vi "Teleop.vi"(10 "Match Info":T7={"Autonomous Elapsed Seconds"=0.0, "TeleOp Elapsed Seconds"=0.0, "Disabled Elapsed Seconds"=0.0, "Visited Autonomous"=FALSE, "Visited TeleOp"=FALSE, "Visited Disabled"=FALSE, "Autonomous Settings"={"Autonomous Style"=enum."Independent", "VI Refnum"=refnum}}, 11 "Call Context":T8) -> ()   [LabVIEW 2018]
doc: "This VI is called for each TeleOp packet received from the DS where the robot is not disabled. It is often used to read from the joysticks and update I/O or to update setpoints for timed control loops. It should complete and return within 20 milliseconds or it may miss DS packets."
uses:
  <vilib>/Rock Robotics/WPI/DriverStation/WPI_DriverStationDerivedRobotMode.ctl
  <vilib>/Rock Robotics/WPI/DriverStation/WPI_DriverStationMatch Info.ctl
  <vilib>/Rock Robotics/WPI/ThirdParty/Phoenix-LabVIEW/Motor Controller/Controls/CTRE_Phoenix_MotorControl_ControlMode.ctl
  <vilib>/Rock Robotics/WPI/Solenoid/WPI_SolenoidValue.ctl
  <vilib>/Rock Robotics/WPI/Utilities/WPI_GetSetVariantRefNum.vi
  <vilib>/Rock Robotics/Network Tables/NT Write Boolean Array.vi
  <vilib>/Rock Robotics/Network Tables/NT Write Numeric Array.vi
  <vilib>/Rock Robotics/Network Tables/NT Read Boolean.vi
  <vilib>/Rock Robotics/Network Tables/NT Read Number.vi
  <vilib>/Rock Robotics/WPI/Solenoid/WPI_SolenoidSetEnum.vi
  <vilib>/Rock Robotics/WPI/ThirdParty/Phoenix-LabVIEW/Motor Controller/Get/CTRE_Phoenix_MotorController_GetSelectedSensorData.vi
  <vilib>/Utility/inputDevices.llb/joystickAcquire.vi
panel:
  in  "Cluster":T1={"Elevator Setpoints"=[0.0, 100000.0, 250000.0, 250000.0, 270000.0, 475000.0, 50000.0], "Wrist Setpoints"=[180000.0, 7600.0, 82000.0, 100000.0, 4000.0, 69000.0, 100000.0, 110000.0, 205000.0], "Horse Drive Setpoints"=[90000.0, 90000.0, 90000.0, 180000.0], "Wrist Gains"={"proportional gain (Kc)"=-1e-05, "integral time (Ti, min)"=0.01, "derivative time (Td, min)"=0.0}, "Wrist Power Limits"={"output high"=0.75, "output low"=-0.75}, "Horse Gains"={"proportional gain (Kc)"=1e-05, "integral time (Ti, min)"=0.02, "derivative time (Td, min)"=0.0}, "Horse Power Limits"={"output high"=0.25, "output low"=-0.25}, "Elevator Gains"={"proportional gain (Kc)"=1e-05, "integral time (Ti, min)"=0.01, "derivative time (Td, min)"=0.0}, "Elevator Power Limits"={"output high"=0.25, "output low"=-0.25}}
  in  "Wrist Manual Power":dbl step=0.05 format="%#_13g"
  in  "Elevator Manual Power":dbl step=0.05 format="%#_13g"
  in  "Elevator Level Select":T2(ring)
  in  "Horse Drive":T3(ring)
  in  "Wrist":T4(ring)
  in  "Climb Mode":bool
  in  "Elevator Switch":bool=TRUE
  in  "Enable Auto":bool=TRUE
  out "Intake Wrist Encoder":i32
  in  "Reset Intake Wrist":bool
  out "Horse Encoder":i32
  in  "Reset Horse Encoder":bool
  in  "Reset Elevator Encoder":bool
  out "Elevator Encoder":i32
  in  "ScoreMode 2":T5(ring)
  in  "Override Vision":bool
  out "element 2":T6
  in  "Butterfly Status":bool
  in  "ScoreMode":T5(ring)
  out "Sample Slider 0":dbl(slide) scale=0.0..5.0
  out "Sample Boolean 1":bool
  out "Sample Boolean 0":bool
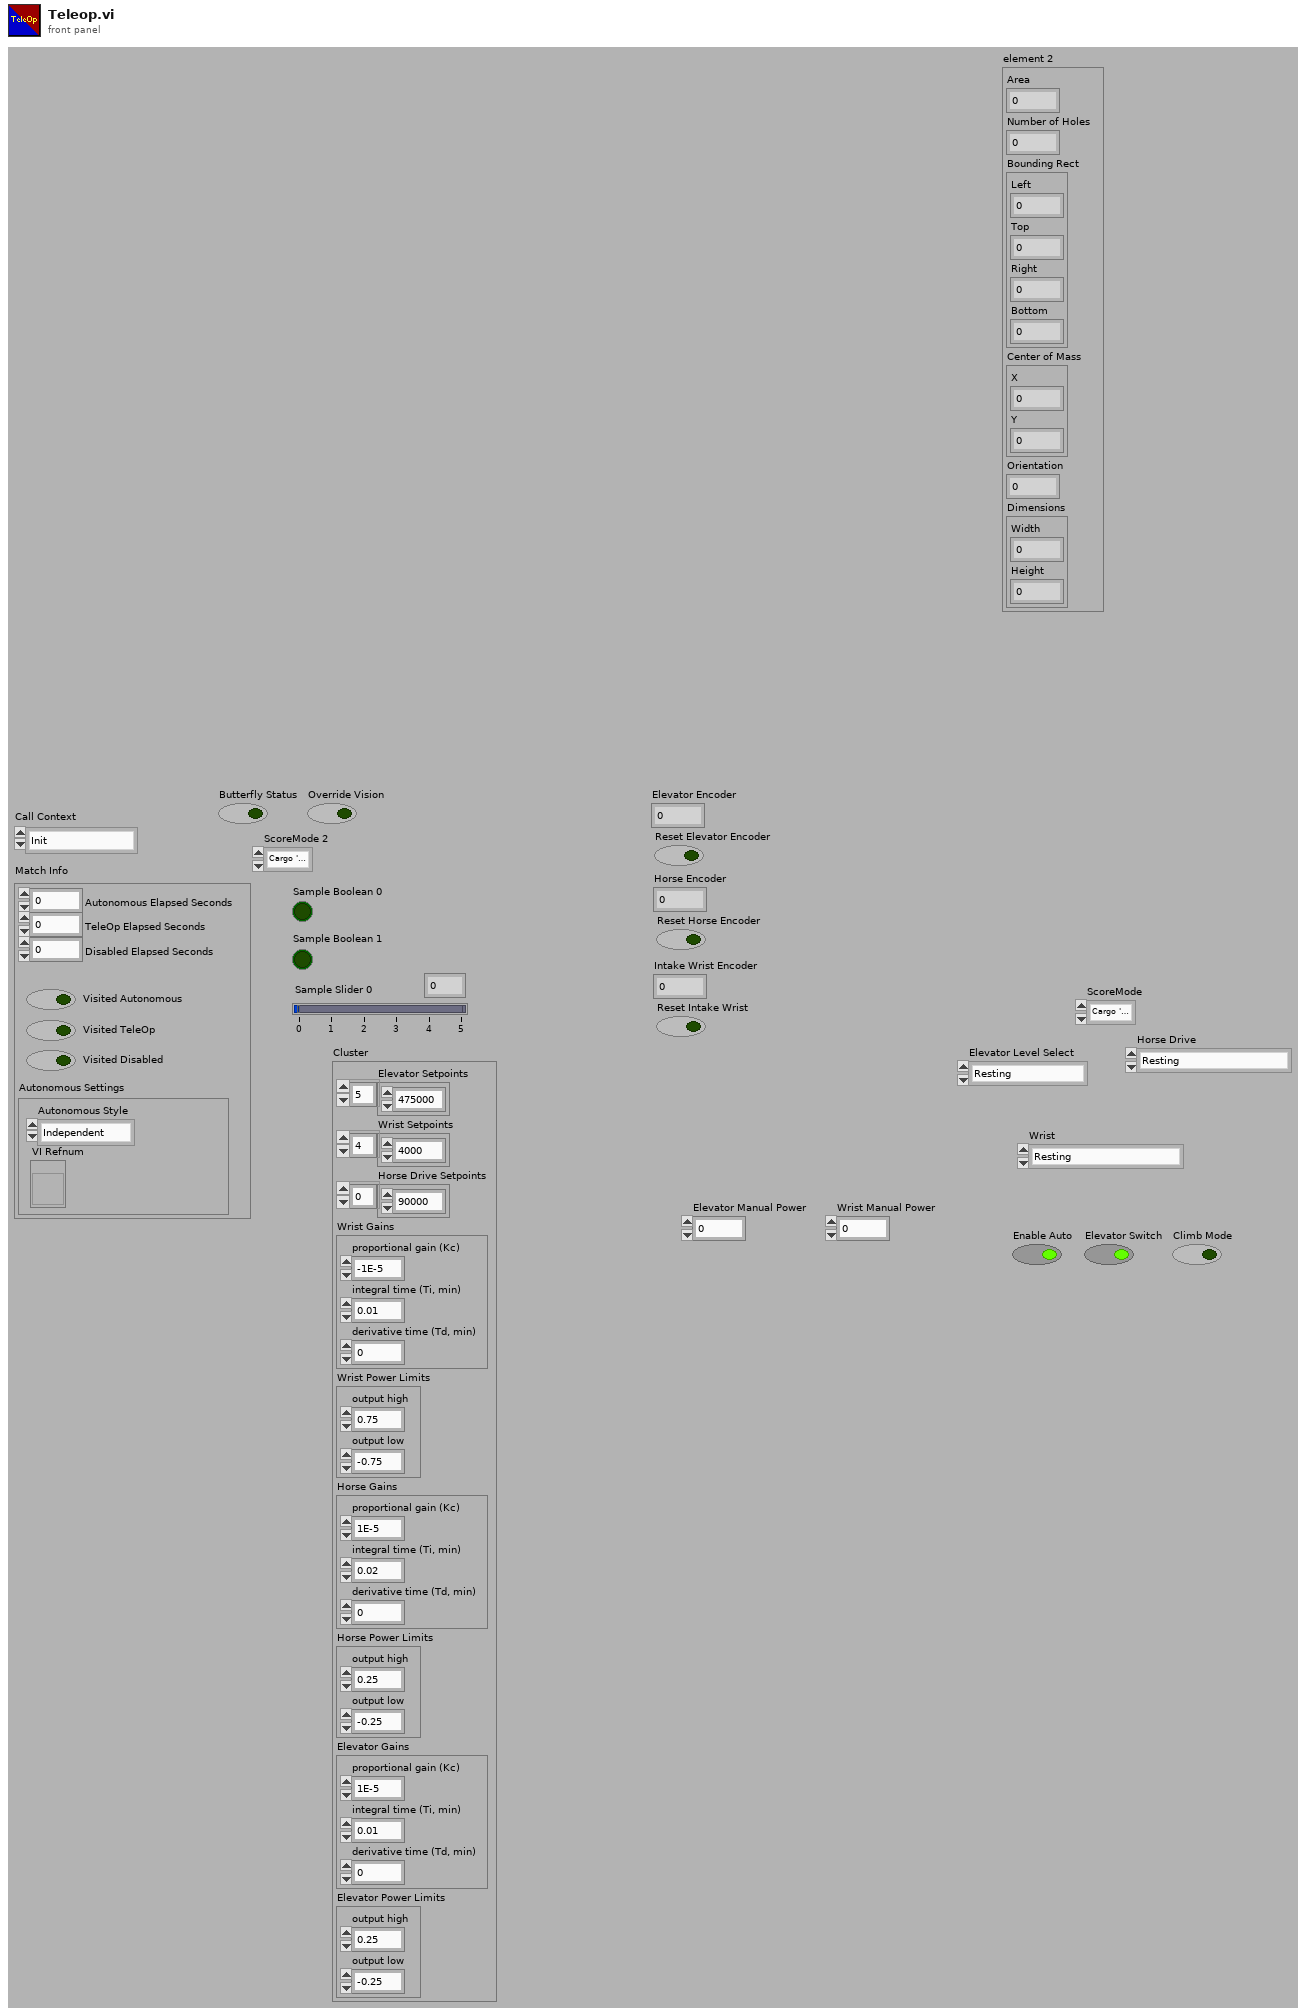
[diagram p1: front panel]
types:
  T1 = cluster{"Elevator Setpoints":dbl[], "Wrist Setpoints":dbl[], "Horse Drive Setpoints":dbl[], "Wrist Gains":cluster{"proportional gain (Kc)":dbl, "integral time (Ti, min)":dbl, "derivative time (Td, min)":dbl}, "Wrist Power Limits":cluster{"output high":dbl, "output low":dbl}, "Horse Gains":cluster{"proportional gain (Kc)":dbl, "integral time (Ti, min)":dbl, "derivative time (Td, min)":dbl}, "Horse Power Limits":cluster{"output high":dbl, "output low":dbl}, "Elevator Gains":cluster{"proportional gain (Kc)":dbl, "integral time (Ti, min)":dbl, "derivative time (Td, min)":dbl}, "Elevator Power Limits":cluster{"output high":dbl, "output low":dbl}}
  T2 = enum16{"Resting", "CargoShip Front", "CargoShip Back", "Cargo Mid", "Hatch Mid", "All High", "Cargo Intake"}
  T3 = enum16{"Resting", "PLACEHOLDER", "Hatch Intake", "Lift"}
  T4 = enum16{"Resting", "Hatch Ground Intake", "Hatch Place Low/Mid/CargoShip", "Hatch Place High", "Cargo Ground Intake", "Cargo Place Low/Mid", "Cargo Place High", "CargoShip Place Front", "CargoShip Place Back"}
  T5 = enum16{"Cargo 'default'", "Hatch", "HorseDriveHatch"}
  T6 = cluster{"Area":dbl, "Number of Holes":dbl, "Bounding Rect":cluster{"Left":dbl, "Top":dbl, "Right":dbl, "Bottom":dbl}, "Center of Mass":cluster{"X":dbl, "Y":dbl}, "Orientation":dbl, "Dimensions":cluster{"Width":dbl, "Height":dbl}}
  T7 = typedef "WPI_DriverStationMatch Info.ctl" = cluster{"Autonomous Elapsed Seconds":dbl, "TeleOp Elapsed Seconds":dbl, "Disabled Elapsed Seconds":dbl, "Visited Autonomous":bool, "Visited TeleOp":bool, "Visited Disabled":bool, "Autonomous Settings":cluster{"Autonomous Style":enum16{"Iterative", "Independent"}, "VI Refnum":refnum<vi>}}
  T8 = typedef "WPI_DriverStationDerivedRobotMode.ctl" = enum16{"Init", "Execute", "Stop"}
  T9 = typedef "WPI_SolenoidValue.ctl" = enum16{"Off", "On", "Forward", "Reverse"}
  T10 = typedef "CTRE_Phoenix_MotorControl_ControlMode.ctl" = u16
  T11 = typedef "WPI_SolenoidDevRef.ctl" = cluster{"DevStatus":errorcluster, "Pneumatics Control Module":u8, "Forward Solenoid Channel":T12, "Reverse Solenoid Channel":T12}
  T12 = typedef "WPI_SolenoidChannel.ctl" = enum8{"Solenoid 0", "Solenoid 1", "Solenoid 2", "Solenoid 3", "Solenoid 4", "Solenoid 5", "Solenoid 6", "Solenoid 7", "Invalid"}
  T13 = typedef "WPI_JoystickDevRef.ctl" = cluster{"Device":T14}
  T14 = typedef "WPI_JoystickDeviceEnum.ctl" = enum16{"USB 0", "USB 1", "USB 2", "USB 3", "USB 4", "USB 5"}
  T15 = typedef "WPI_MotorControlDeviceRef.ctl" = cluster{"DeviceStatus":errorcluster, "Type":T16, "PWM":cluster{"PWM Channel":T17, "DeadBand":T18}, "CAN":cluster{"Device Number":u8, "SetOutput VI Ref":variant, "GetOutput VI Ref":variant, "Enable VI Ref":variant, "Disable VI Ref":variant, "Data":variant}, "Invert":bool, "DIO PWM":cluster{"PWM \"Enable\" Channel":T17, "DIOChannel":T19, "PWM Rate":dbl}}
  T16 = typedef "WPI_MotorControlType.ctl" = enum16{"PWM", "CAN", "DIO PWM"}
  T17 = typedef "FPGA_DIOPWMChannel.ctl" = enum8{"PWM 0", "PWM 1", "PWM 2", "PWM 3", "PWM 4", "PWM 5", "PWM 6", "PWM 7", "PWM 8", "PWM 9", "PWM MXP 0", "PWM MXP 1", "PWM MXP 2", "PWM MXP 3", "PWM MXP 4", "PWM MXP 5", "PWM MXP 6", "PWM MXP 7", "PWM MXP 8", "PWM MXP 9", "Invalid"}
  T18 = typedef "WPI_PWMDeadband.ctl" = cluster{"Name":string, "maxPositivePwm":i32, "minPositivePwm":i32, "centerPwm":i32, "maxNegativePwm":i32, "minNegativePwm":i32, "angularRange":u16}
  T19 = typedef "FPGA_DIOChannel.ctl" = enum8{"DIO 0", "DIO 1", "DIO 2", "DIO 3", "DIO 4", "DIO 5", "DIO 6", "DIO 7", "DIO 8", "DIO 9", "DIO MXP 0", "DIO MXP 1", "DIO MXP 2", "DIO MXP 3", "DIO MXP 4", "DIO MXP 5", "DIO MXP 6", "DIO MXP 7", "DIO MXP 8", "DIO MXP 9", "DIO MXP 10", "DIO MXP 11", "DIO MXP 12", "DIO MXP 13", "DIO MXP 14", "DIO MXP 15", "SPI Port CS1", "SPI Port CS2", "SPI Port CS3", "SPI Port MISO", "SPI Port MOSI", "Invalid"}
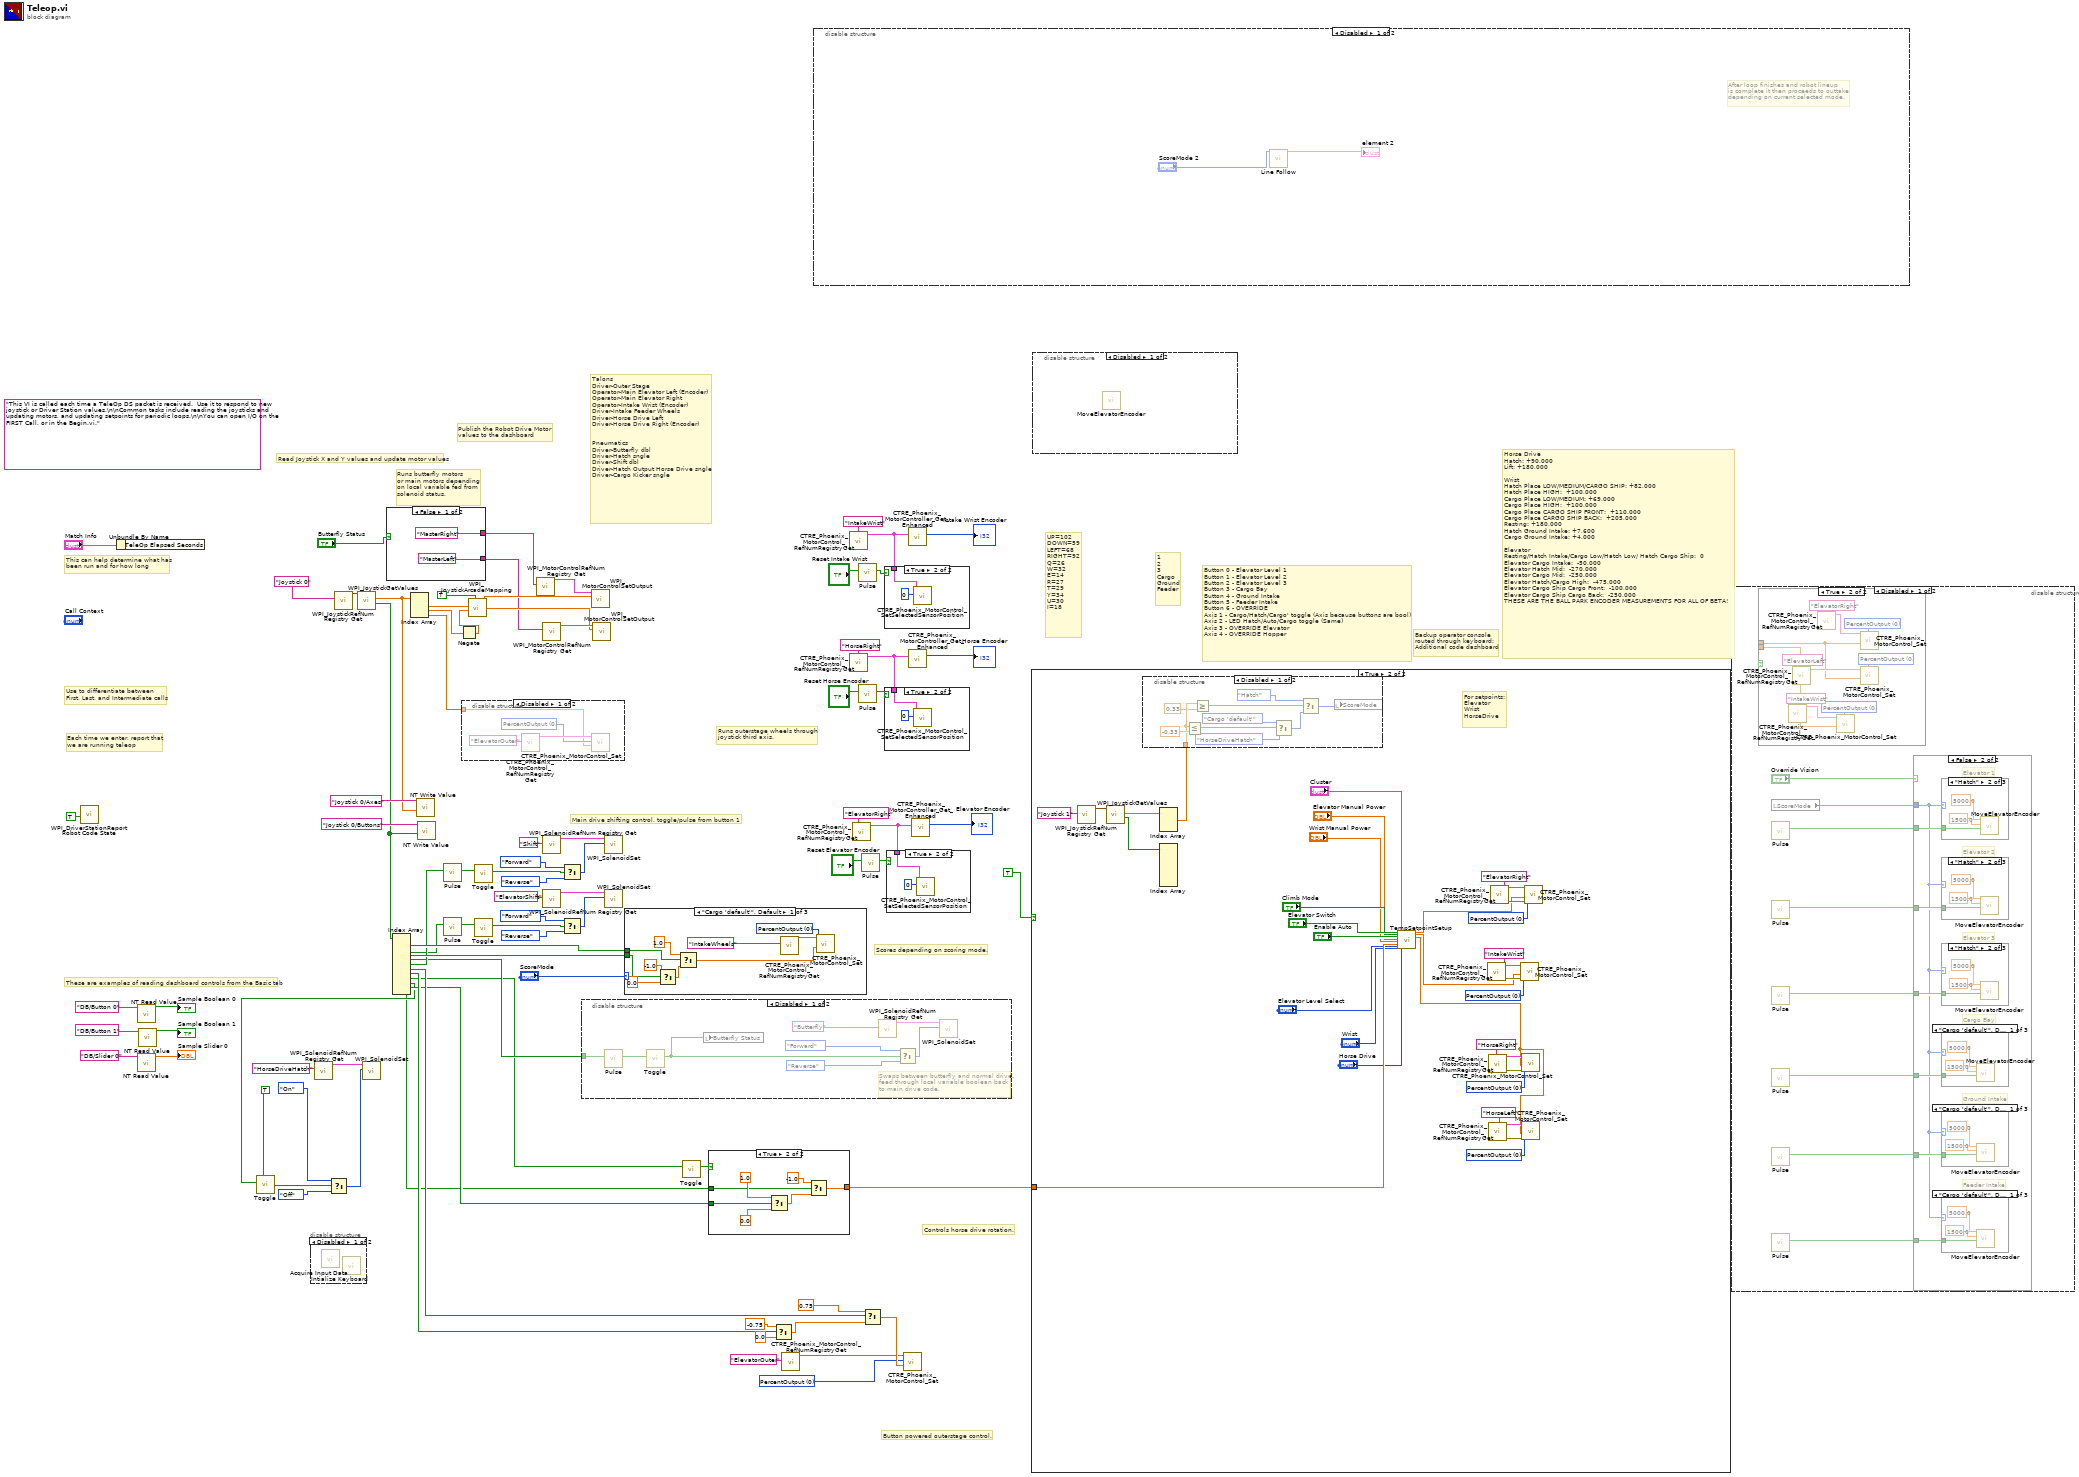
[diagram p0: block diagram]
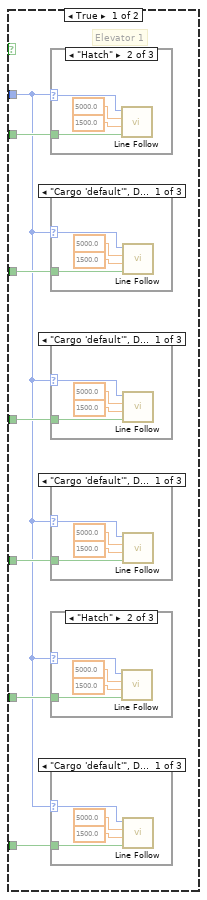
[diagram p3: hidden frame]
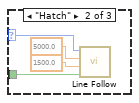
[diagram p4: hidden frame]
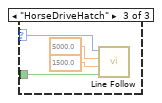
[diagram p5: hidden frame]
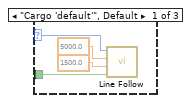
[diagram p6: hidden frame]
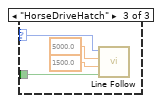
[diagram p7: hidden frame]
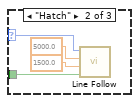
[diagram p8: hidden frame]
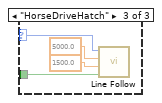
[diagram p9: hidden frame]
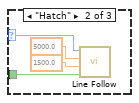
[diagram p10: hidden frame]
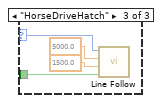
[diagram p11: hidden frame]
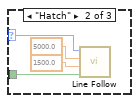
[diagram p12: hidden frame]
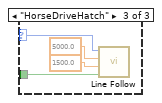
[diagram p13: hidden frame]
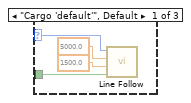
[diagram p14: hidden frame]
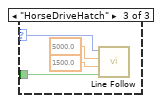
[diagram p15: hidden frame]
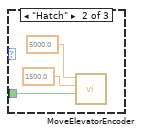
[diagram p16: hidden frame]
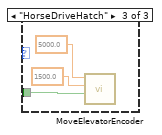
[diagram p17: hidden frame]
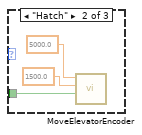
[diagram p18: hidden frame]
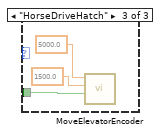
[diagram p19: hidden frame]
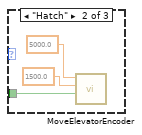
[diagram p20: hidden frame]
diagram:
  w54 = T10 0 items=["PercentOutput"=0, "Position"=1, "Velocity"=2, "Current"=3, "Follower"=5, "MotionProfile"=6, "MotionMagic"=7, "MotionProfileArc"=10, "Disabled"=15] ("Control Mode")
  (unwired) "This VI is called each time a TeleOp DS packet is received.  Use it to respond to new joystick or Driver Station values.\n\nCommon tasks include reading the joysticks and updating motors, and updating setpoints for periodic loops.\n\nYou can open I/O on the FIRST Call, or in the Begin.vi."
  # "Horse Drive\nHatch: +90,000\nLift: +180,000\n\nWrist\nHatch Place LOW/MEDIUM/CARGO SHIP: +82,000\nHatch Place HIGH:  +100,000\nCargo Place LOW/MEDIUM: +69,000\nCargo Place HIGH:  +100,000\nCargo Place CARGO SHIP FRONT:  +110,000\nCargo Place CARGO SHIP BACK:  +205,000\nResting: +180,000\nHatch Ground Intake: +7,600\nCargo Ground Intake: +4,000\n\nElevator\nResting/Hatch Intake/Cargo Low/Hatch Low/ Hatch Cargo Ship:  0\nElevator Cargo Intake:  -50,000\nElevator Hatch Mid:  -270,000\nElevator Cargo Mid:  -250,000\nElevator Hatch/Cargo High:  -475,000\nElevator Cargo Ship Cargo Front:  -100,000\nElevator Cargo Ship Cargo Back:  -250,000\nTHESE ARE THE BALL PARK ENCODER MEASUREMENTS FOR ALL OF BETA!"
  # "Button 0 - Elevator Level 1\nButton 1 - Elevator Level 2\nButton 2 - Elevator Level 3\nButton 3 - Cargo Bay\nButton 4 - Ground Intake\nButton 5 - Feeder Intake\nButton 6 - OVERRIDE\nAxis 1 - Cargo/Hatch/Cargo' toggle (Axis because buttons are bool)\nAxis 2 - LED Hatch/Auto/Cargo toggle (Same)\nAxis 3 - OVERRIDE Elevator\nAxis 4 - OVERRIDE Hopper"
  # "1\n2\n3\nCargo\nGround\nFeeder"
  # "Button powered outerstage control."
  # "Controls horse drive rotation."
  # "Scores depending on scoring mode."
  # "Main drive shifting control, toggle/pulse from button 1"
  # "Runs outerstage wheels through\njoystick third axis."
  # "Runs butterfly motors\nor main motors depending\non local variable fed from\nsolenoid status."
  # "Backup operator console\nrouted through keyboard:\nAdditional code dashboard"
  # "UP=102\nDOWN=59\nLEFT=68\nRIGHT=92\nQ=26\nW=32\nE=14\nR=27\nT=29\nY=34\nU=30\nI=18"
  # "Talons\nDriver-Outer Stage \nOperator-Main Elevator Left (Encoder)\nOperator-Main Elevator Right\nOperator-Intake Wrist (Encoder)\nDriver-Intake Feeder Wheels\nDriver-Horse Drive Left\nDriver-Horse Drive Right (Encoder)\n\n\nPneumatics\nDriver-Butterfly dbl \nDriver-Hatch sngle\nDriver-Shift dbl\nDriver-Hatch Output Horse Drive sngle\nDriver-Cargo Kicker sngle"
  # "These are examples of reading dashboard controls from the Basic tab"
  # "Publish the Robot Drive Motor\nvalues to the dashboard"
  # "Each time we enter, report that\nwe are running teleop"
  # "Use to differentiate between\nFirst, Last, and Intermediate calls"
  # "This can help determine what has\nbeen run and for how long"
  # "Read Joystick X and Y values and update motor values"
  n1 = call <vilib>:"WPI_DriverStationReport Robot Code State.vi"("TeleOp"=TRUE ("Autonomous")) -> ()  [unwired: 10 in, 1 out]
  n2 = Unbundle By Name("Match Info") -> ()  [unwired: 1 out]
  n3 = call-poly <vilib>:"NT Read Value.vi"("Name"="DB/Button 0" ("refnum name")) -> ("Boolean"=→"Sample Boolean 0":bool)  [unwired: 9 in, 1 out]
  n4 = call-poly <vilib>:"NT Read Value.vi"("Name"="DB/Slider 0" ("refnum name")) -> ("Numeric"=→"Sample Slider 0":dbl)  [unwired: 9 in, 1 out]
  n5 = call-poly <vilib>:"NT Read Value.vi"("Name"="DB/Button 1" ("refnum name")) -> ("Boolean"=→"Sample Boolean 1":bool)  [unwired: 9 in, 1 out]
  n6 = disable-structure shown="Disabled" {
    frame Disabled {
      n7 = call-poly <vilib>:"Acquire Input Data.vi"() -> ()  [unwired: 15 in, 5 out]
      n8 = call <vilib>:"Intialize Keyboard.vi"() -> ()  [unwired: 10 in, 2 out]
    }
    frame Enabled {
    }
  }
  n9 = call <vilib>:"WPI_SolenoidRefNum Registry Get.vi"("refnum name"="HorseDriveHatch") -> ("SolenoidDevRef"=w22:T11)  [unwired: 9 in, 1 out]
  n10 = call <vilib>:"WPI_JoystickRefNum Registry Get.vi"("refnum name"="Joystick 0") -> ("JoystickDevRef"=w83:T13)  [unwired: 1 in, 9 out]
  n11 = call <vilib>:"WPI_JoystickGetValues.vi"("JoystickDevRef"=w83) -> ("Buttons"=w66:bool[], "Axes"=w79:dbl[])  [unwired: 6 in, 3 out]
  n12 = case shown="False" "Butterfly Status" {
    tunnel: ["MasterRight" ("refnum name") "spark4" ("refnum name")] -> w46
    tunnel: ["MasterLeft" ("refnum name") "spark5" ("refnum name")] -> w45
    frame False {
    }
    frame True {
    }
  }
  n13 = Index Array(array=w66) -> (element #1=w43:bool, element #2=w33:bool, element #3=w58:bool, element #4=w41:bool, element #5=w42:bool, element #6=w32:bool, element #7=w31:bool, element #8=w3:bool, element #9=w25:bool, element #10=w30:bool, element #11=w2:bool)  [unwired: 11 in]
  n14 = call "Toggle.vi"("Control"=TRUE, "Input"=w25) -> ("Output"=w24:bool)  [unwired: 9 in]
  n15 = Select(t=WPI_SolenoidValue."On" ("Value"), s=w24, f=WPI_SolenoidValue."Off" ("Value")) -> (s? t:f=w29:T9)
  n16 = call-poly <vilib>:"WPI_SolenoidSet.vi"("Value"=w29, "SolenoidDevRef"=w22) -> ()  [unwired: 8 in, 2 out]
  n17 = Index Array(array=w79) -> (element #1=w72:dbl, element #2=w6:dbl, element #3=w47:dbl)  [unwired: 3 in]
  n18 = call-poly <vilib>:"NT Write Value.vi"("Numeric Array"=w79, "Name"="Joystick 0/Axes") -> ()  [unwired: 9 in, 1 out]
  n19 = call-poly <vilib>:"NT Write Value.vi"("Boolean Array"=w66, "Name"="Joystick 0/Buttons") -> ()  [unwired: 9 in, 1 out]
  n20 = call "Pulse.vi"("Input"=w42) -> ("Output"=w61:bool)  [unwired: 10 in]
  n21 = call "Pulse.vi"("Input"=w33) -> ("Output"=w38:bool)  [unwired: 10 in]
  n22 = Negate(x=w6) -> (-x=w5:dbl)
  n23 = disable-structure shown="Disabled" {
    disable-tunnel: w47 -> [w90 _]
    frame Disabled {
      w91 = T10 0 items=["PercentOutput"=0, "Position"=1, "Velocity"=2, "Current"=3, "Follower"=5, "MotionProfile"=6, "MotionMagic"=7, "MotionProfileArc"=10, "Disabled"=15] ("Control Mode")
      n24 = call <vilib>:"CTRE_Phoenix_MotorControl_RefNumRegistryGet.vi"("refnum name"="ElevatorOuter") -> ("PhoenixMotorControlDevRef"=w92:T15)  [unwired: 9 in, 1 out]
      n25 = call <vilib>:"CTRE_Phoenix_MotorControl_Set.vi"("Output"=w90, "Control Mode"=w91, "PhoenixMotorControlDevRef"=w92) -> ()  [unwired: 7 in, 2 out]
    }
    frame Enabled {
    }
  }
  n26 = call <vilib>:"WPI_JoystickArcadeMapping.vi"("Square Inputs"=TRUE, "Y axis value"=w5, "X axis value"=w72) -> ("Right Motor Value"=w67:dbl, "Left Motor Value"=w69:dbl)  [unwired: 7 in]
  n27 = call "Toggle.vi"("Input"=w61) -> ("Output"=w60:bool)  [unwired: 10 in]
  n28 = call "Toggle.vi"("Input"=w38) -> ("Output"=w39:bool)  [unwired: 10 in]
  n29 = call <vilib>:"WPI_MotorControlRefNum Registry Get.vi"("refnum name"=w46) -> ("MotorControlDevRef"=w70:T15)  [unwired: 9 in, 1 out]
  n30 = call <vilib>:"WPI_MotorControlRefNum Registry Get.vi"("refnum name"=w45) -> ("MotorControlDevRef"=w68:T15)  [unwired: 9 in, 1 out]
  n31 = call <vilib>:"WPI_SolenoidRefNum Registry Get.vi"("refnum name"="Shift") -> ("SolenoidDevRef"=w64:T11)  [unwired: 9 in, 1 out]
  n32 = call <vilib>:"WPI_SolenoidRefNum Registry Get.vi"("refnum name"="ElevatorShift") -> ("SolenoidDevRef"=w35:T11)  [unwired: 9 in, 1 out]
  n33 = Select(t=WPI_SolenoidValue."Forward" ("Value"), s=w60, f=WPI_SolenoidValue."Reverse" ("Value")) -> (s? t:f=w59:T9)
  n34 = Select(t=WPI_SolenoidValue."Forward" ("Value"), s=w39, f=WPI_SolenoidValue."Reverse" ("Value")) -> (s? t:f=w40:T9)
  n35 = disable-structure shown="Disabled" {
    disable-tunnel: w41 -> [w94 _]
    frame Disabled {
      # "Swaps between butterfly and normal drive,\nfeed through local variable boolean back\nto main drive code."
      n36 = call "Pulse.vi"("Input"=w94) -> ("Output"=w101:bool)  [unwired: 10 in]
      n37 = call "Toggle.vi"("Input"=w101) -> ("Output"=w95:bool)  [unwired: 10 in]
      n38 = local write "Butterfly Status"(w95) -> ()
      n39 = call <vilib>:"WPI_SolenoidRefNum Registry Get.vi"("refnum name"="Butterfly") -> ("SolenoidDevRef"=w97:T11)  [unwired: 9 in, 1 out]
      n40 = Select(t=WPI_SolenoidValue."Forward" ("Value"), s=w95, f=WPI_SolenoidValue."Reverse" ("Value")) -> (s? t:f=w100:T9)
      n41 = call-poly <vilib>:"WPI_SolenoidSet.vi"("Value"=w100, "SolenoidDevRef"=w97) -> ()  [unwired: 8 in, 2 out]
    }
    frame Enabled {
    }
  }
  n42 = call <vilib>:"WPI_MotorControlSetOutput.vi"("Output"=w69, "MotorControlDevRef"=w70) -> ()  [unwired: 7 in, 3 out]
  n43 = call <vilib>:"WPI_MotorControlSetOutput.vi"("Output"=w67, "MotorControlDevRef"=w68) -> ()  [unwired: 7 in, 3 out]
  n44 = call-poly <vilib>:"WPI_SolenoidSet.vi"("Value"=w59, "SolenoidDevRef"=w64) -> ()  [unwired: 8 in, 2 out]
  n45 = call-poly <vilib>:"WPI_SolenoidSet.vi"("Value"=w40, "SolenoidDevRef"=w35) -> ()  [unwired: 8 in, 2 out]
  n46 = case shown="\"Cargo 'default'\", Default" "ScoreMode" {
    tunnel: w43 -> [w108 w117 w126]
    tunnel: w58 -> [w107 w118 w127]
    frame "Cargo 'default'", Default {
      w109 = T10 0 items=["PercentOutput"=0, "Position"=1, "Velocity"=2, "Current"=3, "Follower"=5, "MotionProfile"=6, "MotionMagic"=7, "MotionProfileArc"=10, "Disabled"=15] ("Control Mode")
      n47 = Select(t=-1.0, s=w107, f=0.0) -> (s? t:f=w106:dbl)
      n48 = Select(t=1.0, s=w108, f=w106) -> (s? t:f=w102:dbl)
      n49 = call <vilib>:"CTRE_Phoenix_MotorControl_RefNumRegistryGet.vi"("refnum name"="IntakeWheels") -> ("PhoenixMotorControlDevRef"=w110:T15)  [unwired: 9 in, 1 out]
      n50 = call <vilib>:"CTRE_Phoenix_MotorControl_Set.vi"("Output"=w102, "Control Mode"=w109, "PhoenixMotorControlDevRef"=w110) -> ()  [unwired: 7 in, 2 out]
    }
    frame "HorseDriveHatch" {
      n51 = Or(x=w117, y=w118) -> (x .or. y?=w116:bool)
      n52 = call "Pulse.vi"("Input"=w116) -> ("Output"=w112:bool)  [unwired: 10 in]
      n53 = call <vilib>:"WPI_SolenoidRefNum Registry Get.vi"("refnum name"="HorseDriveHatch") -> ("SolenoidDevRef"=w120:T11)  [unwired: 9 in, 1 out]
      n54 = Select(t=WPI_SolenoidValue."On" ("Value"), s=w112, f=WPI_SolenoidValue."Off" ("Value")) -> (s? t:f=w113:T9)
      n55 = call-poly <vilib>:"WPI_SolenoidSet.vi"("Value"=w113, "SolenoidDevRef"=w120) -> ()  [unwired: 8 in, 2 out]
    }
    frame "Hatch" {
      n56 = Or(x=w126, y=w127) -> (x .or. y?=w125:bool)
      n57 = call "Pulse.vi"("Input"=w125) -> ("Output"=w121:bool)  [unwired: 10 in]
      n58 = call <vilib>:"WPI_SolenoidRefNum Registry Get.vi"("refnum name"="Hatch") -> ("SolenoidDevRef"=w129:T11)  [unwired: 9 in, 1 out]
      n59 = Select(t=WPI_SolenoidValue."On" ("Value"), s=w121, f=WPI_SolenoidValue."Off" ("Value")) -> (s? t:f=w122:T9)
      n60 = call-poly <vilib>:"WPI_SolenoidSet.vi"("Value"=w122, "SolenoidDevRef"=w129) -> ()  [unwired: 8 in, 2 out]
    }
  }
  n61 = call "Toggle.vi"("Input"=w3) -> ("Output"=w4:bool)  [unwired: 10 in]
  n62 = case shown="True" w4 {
    tunnel: [w131 w141] -> w1
    tunnel: w30 -> [w132 w140]
    tunnel: w2 -> [w130 w137]
    frame False {
      n63 = Select(t=0.4, s=w132, f=0.0) -> (s? t:f=w136:dbl)
      n64 = Select(t=-0.2, s=w130, f=w136) -> (s? t:f=w131:dbl)
    }
    frame True {
      n65 = Select(t=1.0, s=w140, f=0.0) -> (s? t:f=w143:dbl)
      n66 = Select(t=-1.0, s=w137, f=w143) -> (s? t:f=w141:dbl)
    }
  }
  n67 = Select(t=-0.75, s=w31, f=0.0) -> (s? t:f=w48:dbl)
  n68 = call <vilib>:"CTRE_Phoenix_MotorControl_RefNumRegistryGet.vi"("refnum name"="ElevatorOuter") -> ("PhoenixMotorControlDevRef"=w53:T15)  [unwired: 9 in, 1 out]
  n69 = disable-structure shown="Disabled" {
    frame Disabled {
      # "After loop finishes and robot lineup\nis complete it then proceeds to outtake\ndepending on current selected mode."
      n70 = call "Line Follow.vi"("ScoreMode in"="ScoreMode 2") -> ("element 2"=→"element 2":T6)  [unwired: 10 in]
    }
    frame Enabled {
    }
  }
  n71 = call <vilib>:"CTRE_Phoenix_MotorControl_RefNumRegistryGet.vi"("refnum name"="IntakeWrist") -> ("PhoenixMotorControlDevRef"=w10:T15)  [unwired: 9 in, 1 out]
  n72 = call <vilib>:"CTRE_Phoenix_MotorControl_RefNumRegistryGet.vi"("refnum name"="HorseRight") -> ("PhoenixMotorControlDevRef"=w16:T15)  [unwired: 9 in, 1 out]
  n73 = call <vilib>:"CTRE_Phoenix_MotorControl_RefNumRegistryGet.vi"("refnum name"="ElevatorRight") -> ("PhoenixMotorControlDevRef"=w19:T15)  [unwired: 9 in, 1 out]
  n74 = call "Pulse.vi"("Input"="Reset Intake Wrist") -> ("Output"=w7:bool)  [unwired: 10 in]
  n75 = call "Pulse.vi"("Input"="Reset Horse Encoder") -> ("Output"=w15:bool)  [unwired: 10 in]
  n76 = call "Pulse.vi"("Input"="Reset Elevator Encoder") -> ("Output"=w20:bool)  [unwired: 10 in]
  n77 = Select(t=0.75, s=w32, f=w48) -> (s? t:f=w55:dbl)
  n78 = case shown="True" w7 {
    tunnel: w10 -> [_ w147]
    frame False {
    }
    frame True {
      n79 = call <vilib>:"CTRE_Phoenix_MotorControl_SetSelectedSensorPosition.vi"("New Sensor Position"=0, "PhoenixMotorControlDevRef"=w147) -> ()  [unwired: 8 in, 2 out]
    }
  }
  n80 = case shown="True" w15 {
    tunnel: w16 -> [_ w149]
    frame False {
    }
    frame True {
      n81 = call <vilib>:"CTRE_Phoenix_MotorControl_SetSelectedSensorPosition.vi"("New Sensor Position"=0, "PhoenixMotorControlDevRef"=w149) -> ()  [unwired: 8 in, 2 out]
    }
  }
  n82 = case shown="True" w20 {
    tunnel: w19 -> [_ w151]
    frame False {
    }
    frame True {
      n83 = call <vilib>:"CTRE_Phoenix_MotorControl_SetSelectedSensorPosition.vi"("New Sensor Position"=0, "PhoenixMotorControlDevRef"=w151) -> ()  [unwired: 8 in, 2 out]
    }
  }
  n84 = call <vilib>:"CTRE_Phoenix_MotorControl_Set.vi"("Output"=w55, "Control Mode"=w54, "PhoenixMotorControlDevRef"=w53) -> ()  [unwired: 7 in, 2 out]
  n85 = call-poly <vilib>:"CTRE_Phoenix_MotorController_Get_Enhanced.vi"("PhoenixMotorControlDevRef"=w10) -> ("Position (Raw Sensor Units)"=→"Intake Wrist Encoder":i32)  [unwired: 11 in, 3 out]
  n86 = call-poly <vilib>:"CTRE_Phoenix_MotorController_Get_Enhanced.vi"("PhoenixMotorControlDevRef"=w16) -> ("Position (Raw Sensor Units)"=→"Horse Encoder":i32)  [unwired: 11 in, 3 out]
  n87 = call-poly <vilib>:"CTRE_Phoenix_MotorController_Get_Enhanced.vi"("PhoenixMotorControlDevRef"=w19) -> ("Position (Raw Sensor Units)"=→"Elevator Encoder":i32)  [unwired: 11 in, 3 out]
  n88 = case shown="True" TRUE {
    tunnel: w1 -> [_ w290]
    frame False {
      n89 = call-poly <vilib>:"NT Read Value.vi"("Default Value"=0.0, "Name"="Keyboard Data") -> ("Numeric"=w152:dbl)  [unwired: 8 in, 1 out]
      n90 = case shown="92" w152 {
        frame 0, Default {
          w158 = 0.0 ("Output")
          w155 = T10 0 items=["PercentOutput"=0, "Position"=1, "Velocity"=2, "Current"=3, "Follower"=5, "MotionProfile"=6, "MotionMagic"=7, "MotionProfileArc"=10, "Disabled"=15] ("Control Mode")
          w157 = T10 0 items=["PercentOutput"=0, "Position"=1, "Velocity"=2, "Current"=3, "Follower"=5, "MotionProfile"=6, "MotionMagic"=7, "MotionProfileArc"=10, "Disabled"=15] ("Control Mode")
          w165 = T10 0 items=["PercentOutput"=0, "Position"=1, "Velocity"=2, "Current"=3, "Follower"=5, "MotionProfile"=6, "MotionMagic"=7, "MotionProfileArc"=10, "Disabled"=15] ("Control Mode")
          n91 = call <vilib>:"CTRE_Phoenix_MotorControl_RefNumRegistryGet.vi"("refnum name"="ElevatorLeft") -> ("PhoenixMotorControlDevRef"=w161:T15)  [unwired: 9 in, 1 out]
          n92 = call <vilib>:"CTRE_Phoenix_MotorControl_RefNumRegistryGet.vi"("refnum name"="ElevatorRight") -> ("PhoenixMotorControlDevRef"=w160:T15)  [unwired: 9 in, 1 out]
          n93 = call <vilib>:"CTRE_Phoenix_MotorControl_Set.vi"("Output"=w158, "Control Mode"=w157, "PhoenixMotorControlDevRef"=w160) -> ()  [unwired: 7 in, 2 out]
          n94 = call <vilib>:"CTRE_Phoenix_MotorControl_Set.vi"("Output"=w158, "Control Mode"=w155, "PhoenixMotorControlDevRef"=w161) -> ()  [unwired: 7 in, 2 out]
          n95 = call <vilib>:"CTRE_Phoenix_MotorControl_RefNumRegistryGet.vi"("refnum name"="IntakeWrist") -> ("PhoenixMotorControlDevRef"=w164:T15)  [unwired: 9 in, 1 out]
          n96 = call <vilib>:"CTRE_Phoenix_MotorControl_Set.vi"("Output"=0.0, "Control Mode"=w165, "PhoenixMotorControlDevRef"=w164) -> ()  [unwired: 7 in, 2 out]
        }
        frame 102 {
          w166 = 0.75 ("Output")
          w168 = T10 0 items=["PercentOutput"=0, "Position"=1, "Velocity"=2, "Current"=3, "Follower"=5, "MotionProfile"=6, "MotionMagic"=7, "MotionProfileArc"=10, "Disabled"=15] ("Control Mode")
          w172 = T10 0 items=["PercentOutput"=0, "Position"=1, "Velocity"=2, "Current"=3, "Follower"=5, "MotionProfile"=6, "MotionMagic"=7, "MotionProfileArc"=10, "Disabled"=15] ("Control Mode")
          n97 = call <vilib>:"CTRE_Phoenix_MotorControl_RefNumRegistryGet.vi"("refnum name"="ElevatorLeft") -> ("PhoenixMotorControlDevRef"=w169:T15)  [unwired: 9 in, 1 out]
          n98 = call <vilib>:"CTRE_Phoenix_MotorControl_RefNumRegistryGet.vi"("refnum name"="ElevatorRight") -> ("PhoenixMotorControlDevRef"=w171:T15)  [unwired: 9 in, 1 out]
          n99 = call <vilib>:"CTRE_Phoenix_MotorControl_Set.vi"("Output"=w166, "Control Mode"=w172, "PhoenixMotorControlDevRef"=w171) -> ()  [unwired: 7 in, 2 out]
          n100 = call <vilib>:"CTRE_Phoenix_MotorControl_Set.vi"("Output"=w166, "Control Mode"=w168, "PhoenixMotorControlDevRef"=w169) -> ()  [unwired: 7 in, 2 out]
        }
        frame 59 {
          w173 = -0.75 ("Output")
          w175 = T10 0 items=["PercentOutput"=0, "Position"=1, "Velocity"=2, "Current"=3, "Follower"=5, "MotionProfile"=6, "MotionMagic"=7, "MotionProfileArc"=10, "Disabled"=15] ("Control Mode")
          w179 = T10 0 items=["PercentOutput"=0, "Position"=1, "Velocity"=2, "Current"=3, "Follower"=5, "MotionProfile"=6, "MotionMagic"=7, "MotionProfileArc"=10, "Disabled"=15] ("Control Mode")
          n101 = call <vilib>:"CTRE_Phoenix_MotorControl_RefNumRegistryGet.vi"("refnum name"="ElevatorLeft") -> ("PhoenixMotorControlDevRef"=w176:T15)  [unwired: 9 in, 1 out]
          n102 = call <vilib>:"CTRE_Phoenix_MotorControl_RefNumRegistryGet.vi"("refnum name"="ElevatorRight") -> ("PhoenixMotorControlDevRef"=w178:T15)  [unwired: 9 in, 1 out]
          n103 = call <vilib>:"CTRE_Phoenix_MotorControl_Set.vi"("Output"=w173, "Control Mode"=w179, "PhoenixMotorControlDevRef"=w178) -> ()  [unwired: 7 in, 2 out]
          n104 = call <vilib>:"CTRE_Phoenix_MotorControl_Set.vi"("Output"=w173, "Control Mode"=w175, "PhoenixMotorControlDevRef"=w176) -> ()  [unwired: 7 in, 2 out]
        }
        frame 68 {
          w183 = T10 0 items=["PercentOutput"=0, "Position"=1, "Velocity"=2, "Current"=3, "Follower"=5, "MotionProfile"=6, "MotionMagic"=7, "MotionProfileArc"=10, "Disabled"=15] ("Control Mode")
          n105 = call <vilib>:"CTRE_Phoenix_MotorControl_RefNumRegistryGet.vi"("refnum name"="IntakeWrist") -> ("PhoenixMotorControlDevRef"=w182:T15)  [unwired: 9 in, 1 out]
          n106 = call <vilib>:"CTRE_Phoenix_MotorControl_Set.vi"("Output"=-0.25, "Control Mode"=w183, "PhoenixMotorControlDevRef"=w182) -> ()  [unwired: 7 in, 2 out]
        }
        frame 92 {
          w187 = T10 0 items=["PercentOutput"=0, "Position"=1, "Velocity"=2, "Current"=3, "Follower"=5, "MotionProfile"=6, "MotionMagic"=7, "MotionProfileArc"=10, "Disabled"=15] ("Control Mode")
          n107 = call <vilib>:"CTRE_Phoenix_MotorControl_RefNumRegistryGet.vi"("refnum name"="IntakeWrist") -> ("PhoenixMotorControlDevRef"=w186:T15)  [unwired: 9 in, 1 out]
          n108 = call <vilib>:"CTRE_Phoenix_MotorControl_Set.vi"("Output"=0.25, "Control Mode"=w187, "PhoenixMotorControlDevRef"=w186) -> ()  [unwired: 7 in, 2 out]
        }
        frame 1 {
          n109 = local write "ScoreMode"(T5."Cargo 'default'" ("ScoreMode")) -> ()
        }
        frame 2 {
          n110 = local write "ScoreMode"(T5."Hatch" ("ScoreMode")) -> ()
        }
        frame 3 {
          n111 = local write "ScoreMode"(T5."HorseDriveHatch" ("ScoreMode")) -> ()
        }
        frame 26 {
          n112 = disable-structure shown="Disabled" {
            frame Disabled {
              n113 = local read "ScoreMode"() -> (w191:T5)
              n114 = call "Pulse.vi"("Input"=TRUE ("Output")) -> ("Output"=w193:bool)  [unwired: 10 in]
              n115 = case shown="\"Cargo 'default'\", Default" w191 {
                tunnel: w193 -> [w196 w197 w200]
                frame "Cargo 'default'", Default {
                  n116 = call "MoveElevatorEncoder.vi"(9:w196, "WristSetpoint"=1500.0, "ElevatorSetpoint"=5000.0) -> ()  [unwired: 8 in, 1 out]
                }
                frame "Hatch" {
                  n117 = call "MoveElevatorEncoder.vi"(9:w197, "WristSetpoint"=1500.0, "ElevatorSetpoint"=5000.0) -> ()  [unwired: 8 in, 1 out]
                }
                frame "HorseDriveHatch" {
                  n118 = call "MoveElevatorEncoder.vi"(9:w200, "WristSetpoint"=1500.0, "ElevatorSetpoint"=5000.0) -> ()  [unwired: 8 in, 1 out]
                }
              }
            }
            frame Enabled {
            }
          }
        }
        frame 32 {
          n119 = disable-structure shown="Disabled" {
            frame Disabled {
              n120 = local read "ScoreMode"() -> (w203:T5)
              n121 = call "Pulse.vi"("Input"=TRUE ("Output")) -> ("Output"=w205:bool)  [unwired: 10 in]
              n122 = case shown="\"Cargo 'default'\", Default" w203 {
                tunnel: w205 -> [w208 w209 w212]
                frame "Cargo 'default'", Default {
                  n123 = call "MoveElevatorEncoder.vi"(9:w208, "WristSetpoint"=1500.0, "ElevatorSetpoint"=5000.0) -> ()  [unwired: 8 in, 1 out]
                }
                frame "Hatch" {
                  n124 = call "MoveElevatorEncoder.vi"(9:w209, "WristSetpoint"=1500.0, "ElevatorSetpoint"=5000.0) -> ()  [unwired: 8 in, 1 out]
                }
                frame "HorseDriveHatch" {
                  n125 = call "MoveElevatorEncoder.vi"(9:w212, "WristSetpoint"=1500.0, "ElevatorSetpoint"=5000.0) -> ()  [unwired: 8 in, 1 out]
                }
              }
            }
            frame Enabled {
            }
          }
        }
        frame 14 {
          n126 = disable-structure shown="Disabled" {
            frame Disabled {
              n127 = local read "ScoreMode"() -> (w215:T5)
              n128 = call "Pulse.vi"("Input"=TRUE ("Output")) -> ("Output"=w217:bool)  [unwired: 10 in]
              n129 = case shown="\"Cargo 'default'\", Default" w215 {
                tunnel: w217 -> [w220 w221 w224]
                frame "Cargo 'default'", Default {
                  n130 = call "MoveElevatorEncoder.vi"(9:w220, "WristSetpoint"=1500.0, "ElevatorSetpoint"=5000.0) -> ()  [unwired: 8 in, 1 out]
                }
                frame "Hatch" {
                  n131 = call "MoveElevatorEncoder.vi"(9:w221, "WristSetpoint"=1500.0, "ElevatorSetpoint"=5000.0) -> ()  [unwired: 8 in, 1 out]
                }
                frame "HorseDriveHatch" {
                  n132 = call "MoveElevatorEncoder.vi"(9:w224, "WristSetpoint"=1500.0, "ElevatorSetpoint"=5000.0) -> ()  [unwired: 8 in, 1 out]
                }
              }
            }
            frame Enabled {
            }
          }
        }
        frame 27 {
          n133 = disable-structure shown="Disabled" {
            frame Disabled {
              n134 = local read "ScoreMode"() -> (w227:T5)
              n135 = call "Pulse.vi"("Input"=TRUE ("Output")) -> ("Output"=w229:bool)  [unwired: 10 in]
              n136 = case shown="\"Cargo 'default'\", Default" w227 {
                tunnel: w229 -> [w232 w233 w236]
                frame "Cargo 'default'", Default {
                  n137 = call "MoveElevatorEncoder.vi"(9:w232, "WristSetpoint"=1500.0, "ElevatorSetpoint"=5000.0) -> ()  [unwired: 8 in, 1 out]
                }
                frame "Hatch" {
                  n138 = call "MoveElevatorEncoder.vi"(9:w233, "WristSetpoint"=1500.0, "ElevatorSetpoint"=5000.0) -> ()  [unwired: 8 in, 1 out]
                }
                frame "HorseDriveHatch" {
                  n139 = call "MoveElevatorEncoder.vi"(9:w236, "WristSetpoint"=1500.0, "ElevatorSetpoint"=5000.0) -> ()  [unwired: 8 in, 1 out]
                }
              }
            }
            frame Enabled {
            }
          }
        }
        frame 29 {
          n140 = disable-structure shown="Disabled" {
            frame Disabled {
              n141 = local read "ScoreMode 2"() -> (w239:T5)
              n142 = call "Pulse.vi"("Input"=TRUE ("Output")) -> ("Output"=w241:bool)  [unwired: 10 in]
              n143 = case shown="\"Cargo 'default'\", Default" w239 {
                tunnel: w241 -> [w244 w245 w248]
                frame "Cargo 'default'", Default {
                  n144 = call "MoveElevatorEncoder.vi"(9:w244, "WristSetpoint"=1500.0, "ElevatorSetpoint"=5000.0) -> ()  [unwired: 8 in, 1 out]
                }
                frame "Hatch" {
                  n145 = call "MoveElevatorEncoder.vi"(9:w245, "WristSetpoint"=1500.0, "ElevatorSetpoint"=5000.0) -> ()  [unwired: 8 in, 1 out]
                }
                frame "HorseDriveHatch" {
                  n146 = call "MoveElevatorEncoder.vi"(9:w248, "WristSetpoint"=1500.0, "ElevatorSetpoint"=5000.0) -> ()  [unwired: 8 in, 1 out]
                }
              }
            }
            frame Enabled {
            }
          }
        }
        frame 34 {
          n147 = disable-structure shown="Disabled" {
            frame Disabled {
              n148 = local read "ScoreMode"() -> (w251:T5)
              n149 = call "Pulse.vi"("Input"=TRUE ("Output")) -> ("Output"=w253:bool)  [unwired: 10 in]
              n150 = case shown="\"Cargo 'default'\", Default" w251 {
                tunnel: w253 -> [w256 w257 w260]
                frame "Cargo 'default'", Default {
                  n151 = call "MoveElevatorEncoder.vi"(9:w256, "WristSetpoint"=1500.0, "ElevatorSetpoint"=5000.0) -> ()  [unwired: 8 in, 1 out]
                }
                frame "Hatch" {
                  n152 = call "MoveElevatorEncoder.vi"(9:w257, "WristSetpoint"=1500.0, "ElevatorSetpoint"=5000.0) -> ()  [unwired: 8 in, 1 out]
                }
                frame "HorseDriveHatch" {
                  n153 = call "MoveElevatorEncoder.vi"(9:w260, "WristSetpoint"=1500.0, "ElevatorSetpoint"=5000.0) -> ()  [unwired: 8 in, 1 out]
                }
              }
            }
            frame Enabled {
            }
          }
        }
      }
    }
    frame True {
      w264 = T10 0 items=["PercentOutput"=0, "Position"=1, "Velocity"=2, "Current"=3, "Follower"=5, "MotionProfile"=6, "MotionMagic"=7, "MotionProfileArc"=10, "Disabled"=15] ("Control Mode")
      w276 = T10 0 items=["PercentOutput"=0, "Position"=1, "Velocity"=2, "Current"=3, "Follower"=5, "MotionProfile"=6, "MotionMagic"=7, "MotionProfileArc"=10, "Disabled"=15] ("Control Mode")
      w280 = T10 0 items=["PercentOutput"=0, "Position"=1, "Velocity"=2, "Current"=3, "Follower"=5, "MotionProfile"=6, "MotionMagic"=7, "MotionProfileArc"=10, "Disabled"=15] ("Control Mode")
      w281 = T10 0 items=["PercentOutput"=0, "Position"=1, "Velocity"=2, "Current"=3, "Follower"=5, "MotionProfile"=6, "MotionMagic"=7, "MotionProfileArc"=10, "Disabled"=15] ("Control Mode")
      # "For setpoints:\nElevator\nWrist\nHorseDrive"
      n154 = call <vilib>:"WPI_JoystickRefNum Registry Get.vi"("refnum name"="Joystick 1") -> ("JoystickDevRef"=w296:T13)  [unwired: 1 in, 9 out]
      n155 = call <vilib>:"WPI_JoystickGetValues.vi"("JoystickDevRef"=w296) -> ("Buttons"=w293:bool[], "Axes"=w294:dbl[])  [unwired: 6 in, 3 out]
      n156 = Index Array(array=w294) -> (element #1=w292:dbl)  [unwired: 3 in, 2 out]
      n157 = disable-structure shown="Disabled" {
        disable-tunnel: w292 -> [w298 _]
        frame Disabled {
          n158 = Less Or Equal?(x=w298, y=-0.33) -> (x <= y?=w305:bool)
          n159 = Greater Or Equal?(x=w298, y=0.33) -> (x >= y?=w304:bool)
          n160 = Select(t=T5."Cargo 'default'" ("ScoreMode"), s=w305, f=T5."HorseDriveHatch" ("ScoreMode")) -> (s? t:f=w303:T5)
          n161 = Select(t=T5."Hatch" ("ScoreMode"), s=w304, f=w303) -> (s? t:f=w299:T5)
          n162 = local write "ScoreMode"(w299) -> ()
        }
        frame Enabled {
        }
      }
      n163 = Index Array(array=w293) -> ()  [unwired: 7 in, 7 out]
      n164 = call "TempSetpointSetup.vi"("Elevator Switch"="Elevator Switch", "Climb Mode"="Climb Mode", "Enable Auto"="Enable Auto", "Elevator Manual Power"="Elevator Manual Power", "Wrist Manual Power"="Wrist Manual Power", "Horse Drive Manual Power"=w290, "Elevator Level Select"="Elevator Level Select", "Wrist"="Wrist", "Cluster"="Cluster", "Horse Drive"="Horse Drive") -> ("Elevator Power Out"=w272:dbl, "Wrist Power Out"=w271:dbl, "Horse Drive Power Out"=w263:dbl)  [unwired: 15 in]
      n165 = call <vilib>:"CTRE_Phoenix_MotorControl_RefNumRegistryGet.vi"("refnum name"="IntakeWrist") -> ("error out"=w279:errorcluster, "PhoenixMotorControlDevRef"=w278:T15)  [unwired: 9 in]
      n166 = call <vilib>:"CTRE_Phoenix_MotorControl_RefNumRegistryGet.vi"("refnum name"="HorseRight") -> ("error out"=w275:errorcluster, "PhoenixMotorControlDevRef"=w274:T15)  [unwired: 9 in]
      n167 = call <vilib>:"CTRE_Phoenix_MotorControl_RefNumRegistryGet.vi"("refnum name"="HorseLeft") -> ("error out"=w265:errorcluster, "PhoenixMotorControlDevRef"=w266:T15)  [unwired: 9 in]
      n168 = call <vilib>:"CTRE_Phoenix_MotorControl_RefNumRegistryGet.vi"("refnum name"="ElevatorRight") -> ("error out"=w282:errorcluster, "PhoenixMotorControlDevRef"=w283:T15)  [unwired: 9 in]
      n169 = call <vilib>:"CTRE_Phoenix_MotorControl_Set.vi"("error in (no error)"=w279, "Output"=w271, "Control Mode"=w280, "PhoenixMotorControlDevRef"=w278) -> ()  [unwired: 6 in, 2 out]
      n170 = call <vilib>:"CTRE_Phoenix_MotorControl_Set.vi"("error in (no error)"=w275, "Output"=w263, "Control Mode"=w276, "PhoenixMotorControlDevRef"=w274) -> ()  [unwired: 6 in, 2 out]
      n171 = call <vilib>:"CTRE_Phoenix_MotorControl_Set.vi"("error in (no error)"=w265, "Output"=w263, "Control Mode"=w264, "PhoenixMotorControlDevRef"=w266) -> ()  [unwired: 6 in, 2 out]
      n172 = call <vilib>:"CTRE_Phoenix_MotorControl_Set.vi"("error in (no error)"=w282, "Output"=w272, "Control Mode"=w281, "PhoenixMotorControlDevRef"=w283) -> ()  [unwired: 6 in, 2 out]
    }
  }
  n173 = disable-structure shown="Disabled" {
    frame Disabled {
      n174 = call "MoveElevatorEncoder.vi"() -> ()  [unwired: 11 in, 1 out]
    }
    frame Enabled {
    }
  }
  n175 = disable-structure shown="Disabled" {
    frame Disabled {
      n176 = case shown="True" {
        selector: _ -> [_ _]
        tunnel: _ -> [_ w316]
        tunnel: _ -> [_ w315]
        frame False {
        }
        frame True {
          w319 = T10 0 items=["PercentOutput"=0, "Position"=1, "Velocity"=2, "Current"=3, "Follower"=5, "MotionProfile"=6, "MotionMagic"=7, "MotionProfileArc"=10, "Disabled"=15] ("Control Mode")
          w321 = T10 0 items=["PercentOutput"=0, "Position"=1, "Velocity"=2, "Current"=3, "Follower"=5, "MotionProfile"=6, "MotionMagic"=7, "MotionProfileArc"=10, "Disabled"=15] ("Control Mode")
          w325 = T10 0 items=["PercentOutput"=0, "Position"=1, "Velocity"=2, "Current"=3, "Follower"=5, "MotionProfile"=6, "MotionMagic"=7, "MotionProfileArc"=10, "Disabled"=15] ("Control Mode")
          n177 = call <vilib>:"CTRE_Phoenix_MotorControl_RefNumRegistryGet.vi"("refnum name"="IntakeWrist") -> ("PhoenixMotorControlDevRef"=w318:T15)  [unwired: 9 in, 1 out]
          n178 = call <vilib>:"CTRE_Phoenix_MotorControl_RefNumRegistryGet.vi"("refnum name"="ElevatorLeft") -> ("PhoenixMotorControlDevRef"=w322:T15)  [unwired: 9 in, 1 out]
          n179 = call <vilib>:"CTRE_Phoenix_MotorControl_RefNumRegistryGet.vi"("refnum name"="ElevatorRight") -> ("PhoenixMotorControlDevRef"=w324:T15)  [unwired: 9 in, 1 out]
          n180 = call <vilib>:"CTRE_Phoenix_MotorControl_Set.vi"("Output"=w315, "Control Mode"=w319, "PhoenixMotorControlDevRef"=w318) -> ()  [unwired: 7 in, 2 out]
          n181 = call <vilib>:"CTRE_Phoenix_MotorControl_Set.vi"("Output"=w316, "Control Mode"=w325, "PhoenixMotorControlDevRef"=w324) -> ()  [unwired: 7 in, 2 out]
          n182 = call <vilib>:"CTRE_Phoenix_MotorControl_Set.vi"("Output"=w316, "Control Mode"=w321, "PhoenixMotorControlDevRef"=w322) -> ()  [unwired: 7 in, 2 out]
        }
      }
      n183 = local read "ScoreMode"() -> (w313:T5)
      n184 = call "Pulse.vi"() -> ("Output"=w307:bool)  [unwired: 11 in]
      n185 = call "Pulse.vi"() -> ("Output"=w308:bool)  [unwired: 11 in]
      n186 = call "Pulse.vi"() -> ("Output"=w309:bool)  [unwired: 11 in]
      n187 = call "Pulse.vi"() -> ("Output"=w312:bool)  [unwired: 11 in]
      n188 = call "Pulse.vi"() -> ("Output"=w311:bool)  [unwired: 11 in]
      n189 = call "Pulse.vi"() -> ("Output"=w310:bool)  [unwired: 11 in]
      n190 = case shown="False" "Override Vision" {
        tunnel: w307 -> [w332 w411]
        tunnel: w308 -> [w331 w410]
        tunnel: w309 -> [w330 w409]
        tunnel: w310 -> [w327 w408]
        tunnel: w311 -> [w328 w407]
        tunnel: w312 -> [w329 w406]
        tunnel: w313 -> [w326 w405]
        frame True {
          # "Elevator 1"
          n191 = case shown="\"Hatch\"" w326 {
            selector: w326 -> [w394 w400 w402]
            tunnel: w332 -> [w393 w399 w401]
            frame "Cargo 'default'", Default {
              n192 = call "Line Follow.vi"("Initiate"=w393, "WristSetpoint"=1500.0, "ElevatorSetpoint"=5000.0, "ScoreMode in"=w394) -> ()  [unwired: 7 in, 1 out]
            }
            frame "Hatch" {
              n193 = call "Line Follow.vi"("Initiate"=w399, "WristSetpoint"=1500.0, "ElevatorSetpoint"=5000.0, "ScoreMode in"=w400) -> ()  [unwired: 7 in, 1 out]
            }
            frame "HorseDriveHatch" {
              n194 = call "Line Follow.vi"("Initiate"=w401, "WristSetpoint"=1500.0, "ElevatorSetpoint"=5000.0, "ScoreMode in"=w402) -> ()  [unwired: 7 in, 1 out]
            }
          }
          n195 = case shown="\"Cargo 'default'\", Default" w326 {
            selector: w326 -> [w382 w388 w390]
            tunnel: w331 -> [w381 w387 w389]
            frame "Cargo 'default'", Default {
              n196 = call "Line Follow.vi"("Initiate"=w381, "WristSetpoint"=1500.0, "ElevatorSetpoint"=5000.0, "ScoreMode in"=w382) -> ()  [unwired: 7 in, 1 out]
            }
            frame "Hatch" {
              n197 = call "Line Follow.vi"("Initiate"=w387, "WristSetpoint"=1500.0, "ElevatorSetpoint"=5000.0, "ScoreMode in"=w388) -> ()  [unwired: 7 in, 1 out]
            }
            frame "HorseDriveHatch" {
              n198 = call "Line Follow.vi"("Initiate"=w389, "WristSetpoint"=1500.0, "ElevatorSetpoint"=5000.0, "ScoreMode in"=w390) -> ()  [unwired: 7 in, 1 out]
            }
          }
          n199 = case shown="\"Cargo 'default'\", Default" w326 {
            selector: w326 -> [w370 w376 w378]
            tunnel: w330 -> [w369 w375 w377]
            frame "Cargo 'default'", Default {
              n200 = call "Line Follow.vi"("Initiate"=w369, "WristSetpoint"=1500.0, "ElevatorSetpoint"=5000.0, "ScoreMode in"=w370) -> ()  [unwired: 7 in, 1 out]
            }
            frame "Hatch" {
              n201 = call "Line Follow.vi"("Initiate"=w375, "WristSetpoint"=1500.0, "ElevatorSetpoint"=5000.0, "ScoreMode in"=w376) -> ()  [unwired: 7 in, 1 out]
            }
            frame "HorseDriveHatch" {
              n202 = call "Line Follow.vi"("Initiate"=w377, "WristSetpoint"=1500.0, "ElevatorSetpoint"=5000.0, "ScoreMode in"=w378) -> ()  [unwired: 7 in, 1 out]
            }
          }
          n203 = case shown="\"Cargo 'default'\", Default" w326 {
            selector: w326 -> [w358 w364 w366]
            tunnel: w329 -> [w357 w363 w365]
            frame "Cargo 'default'", Default {
              n204 = call "Line Follow.vi"("Initiate"=w357, "WristSetpoint"=1500.0, "ElevatorSetpoint"=5000.0, "ScoreMode in"=w358) -> ()  [unwired: 7 in, 1 out]
            }
            frame "Hatch" {
              n205 = call "Line Follow.vi"("Initiate"=w363, "WristSetpoint"=1500.0, "ElevatorSetpoint"=5000.0, "ScoreMode in"=w364) -> ()  [unwired: 7 in, 1 out]
            }
            frame "HorseDriveHatch" {
              n206 = call "Line Follow.vi"("Initiate"=w365, "WristSetpoint"=1500.0, "ElevatorSetpoint"=5000.0, "ScoreMode in"=w366) -> ()  [unwired: 7 in, 1 out]
            }
          }
          n207 = case shown="\"Hatch\"" w326 {
            selector: w326 -> [w346 w352 w354]
            tunnel: w328 -> [w345 w351 w353]
            frame "Cargo 'default'", Default {
              n208 = call "Line Follow.vi"("Initiate"=w345, "WristSetpoint"=1500.0, "ElevatorSetpoint"=5000.0, "ScoreMode in"=w346) -> ()  [unwired: 7 in, 1 out]
            }
            frame "Hatch" {
              n209 = call "Line Follow.vi"("Initiate"=w351, "WristSetpoint"=1500.0, "ElevatorSetpoint"=5000.0, "ScoreMode in"=w352) -> ()  [unwired: 7 in, 1 out]
            }
            frame "HorseDriveHatch" {
              n210 = call "Line Follow.vi"("Initiate"=w353, "WristSetpoint"=1500.0, "ElevatorSetpoint"=5000.0, "ScoreMode in"=w354) -> ()  [unwired: 7 in, 1 out]
            }
          }
          n211 = case shown="\"Cargo 'default'\", Default" w326 {
            selector: w326 -> [w334 w340 w342]
            tunnel: w327 -> [w333 w339 w341]
            frame "Cargo 'default'", Default {
              n212 = call "Line Follow.vi"("Initiate"=w333, "WristSetpoint"=1500.0, "ElevatorSetpoint"=5000.0, "ScoreMode in"=w334) -> ()  [unwired: 7 in, 1 out]
            }
            frame "Hatch" {
              n213 = call "Line Follow.vi"("Initiate"=w339, "WristSetpoint"=1500.0, "ElevatorSetpoint"=5000.0, "ScoreMode in"=w340) -> ()  [unwired: 7 in, 1 out]
            }
            frame "HorseDriveHatch" {
              n214 = call "Line Follow.vi"("Initiate"=w341, "WristSetpoint"=1500.0, "ElevatorSetpoint"=5000.0, "ScoreMode in"=w342) -> ()  [unwired: 7 in, 1 out]
            }
          }
        }
        frame False {
          # "Feeder Intake"
          # "Ground Intake"
          # "Cargo Bay"
          # "Elevator 3"
          # "Elevator 2"
          # "Elevator 1"
          n215 = case shown="\"Hatch\"" w405 {
            tunnel: w411 -> [w459 w460 w463]
            frame "Cargo 'default'", Default {
              n216 = call "MoveElevatorEncoder.vi"(9:w459, "WristSetpoint"=1500.0, "ElevatorSetpoint"=5000.0) -> ()  [unwired: 8 in, 1 out]
            }
            frame "Hatch" {
              n217 = call "MoveElevatorEncoder.vi"(9:w460, "WristSetpoint"=1500.0, "ElevatorSetpoint"=5000.0) -> ()  [unwired: 8 in, 1 out]
            }
            frame "HorseDriveHatch" {
              n218 = call "MoveElevatorEncoder.vi"(9:w463, "WristSetpoint"=1500.0, "ElevatorSetpoint"=5000.0) -> ()  [unwired: 8 in, 1 out]
            }
          }
          n219 = case shown="\"Hatch\"" w405 {
            tunnel: w410 -> [w450 w451 w454]
            frame "Cargo 'default'", Default {
              n220 = call "MoveElevatorEncoder.vi"(9:w450, "WristSetpoint"=1500.0, "ElevatorSetpoint"=5000.0) -> ()  [unwired: 8 in, 1 out]
            }
            frame "Hatch" {
              n221 = call "MoveElevatorEncoder.vi"(9:w451, "WristSetpoint"=1500.0, "ElevatorSetpoint"=5000.0) -> ()  [unwired: 8 in, 1 out]
            }
            frame "HorseDriveHatch" {
              n222 = call "MoveElevatorEncoder.vi"(9:w454, "WristSetpoint"=1500.0, "ElevatorSetpoint"=5000.0) -> ()  [unwired: 8 in, 1 out]
            }
          }
          n223 = case shown="\"Hatch\"" w405 {
            tunnel: w409 -> [w441 w442 w445]
            frame "Cargo 'default'", Default {
              n224 = call "MoveElevatorEncoder.vi"(9:w441, "WristSetpoint"=1500.0, "ElevatorSetpoint"=5000.0) -> ()  [unwired: 8 in, 1 out]
            }
            frame "Hatch" {
              n225 = call "MoveElevatorEncoder.vi"(9:w442, "WristSetpoint"=1500.0, "ElevatorSetpoint"=5000.0) -> ()  [unwired: 8 in, 1 out]
            }
            frame "HorseDriveHatch" {
              n226 = call "MoveElevatorEncoder.vi"(9:w445, "WristSetpoint"=1500.0, "ElevatorSetpoint"=5000.0) -> ()  [unwired: 8 in, 1 out]
            }
          }
          n227 = case shown="\"Cargo 'default'\", Default" w405 {
            tunnel: w406 -> [w432 w433 w436]
            frame "Cargo 'default'", Default {
              n228 = call "MoveElevatorEncoder.vi"(9:w432, "WristSetpoint"=1500.0, "ElevatorSetpoint"=5000.0) -> ()  [unwired: 8 in, 1 out]
            }
            frame "Hatch" {
              n229 = call "MoveElevatorEncoder.vi"(9:w433, "WristSetpoint"=1500.0, "ElevatorSetpoint"=5000.0) -> ()  [unwired: 8 in, 1 out]
            }
            frame "HorseDriveHatch" {
              n230 = call "MoveElevatorEncoder.vi"(9:w436, "WristSetpoint"=1500.0, "ElevatorSetpoint"=5000.0) -> ()  [unwired: 8 in, 1 out]
            }
          }
          n231 = case shown="\"Cargo 'default'\", Default" w405 {
            tunnel: w407 -> [w423 w424 w427]
            frame "Cargo 'default'", Default {
              n232 = call "MoveElevatorEncoder.vi"(9:w423, "WristSetpoint"=1500.0, "ElevatorSetpoint"=5000.0) -> ()  [unwired: 8 in, 1 out]
            }
            frame "Hatch" {
              n233 = call "MoveElevatorEncoder.vi"(9:w424, "WristSetpoint"=1500.0, "ElevatorSetpoint"=5000.0) -> ()  [unwired: 8 in, 1 out]
            }
            frame "HorseDriveHatch" {
              n234 = call "MoveElevatorEncoder.vi"(9:w427, "WristSetpoint"=1500.0, "ElevatorSetpoint"=5000.0) -> ()  [unwired: 8 in, 1 out]
            }
          }
          n235 = case shown="\"Cargo 'default'\", Default" w405 {
            tunnel: w408 -> [w414 w415 w418]
            frame "Cargo 'default'", Default {
              n236 = call "MoveElevatorEncoder.vi"(9:w414, "WristSetpoint"=1500.0, "ElevatorSetpoint"=5000.0) -> ()  [unwired: 8 in, 1 out]
            }
            frame "Hatch" {
              n237 = call "MoveElevatorEncoder.vi"(9:w415, "WristSetpoint"=1500.0, "ElevatorSetpoint"=5000.0) -> ()  [unwired: 8 in, 1 out]
            }
            frame "HorseDriveHatch" {
              n238 = call "MoveElevatorEncoder.vi"(9:w418, "WristSetpoint"=1500.0, "ElevatorSetpoint"=5000.0) -> ()  [unwired: 8 in, 1 out]
            }
          }
        }
      }
    }
    frame Enabled {
    }
  }
